vi "GetAvgPatientStayTimeMultipleRooms.vi"(8 "error in":errorcluster, 9 "To":timestamp, 10 "From":timestamp, 11 "Rooms":string[](array[string])) -> (0 "error out":errorcluster, 1 "AvgStayTime(s)":dbl, 2 "TotalNumberOfPatients":i32, 3 "AvgStayTimePerRoom":dbl[](array[numeric]), 5 "NumOfPatientsPerRoom":i32[](array[numeric]))   [LabVIEW 2015, in "DatabaseApi.lvlib"]
uses:
  DatabaseApi.lvlib
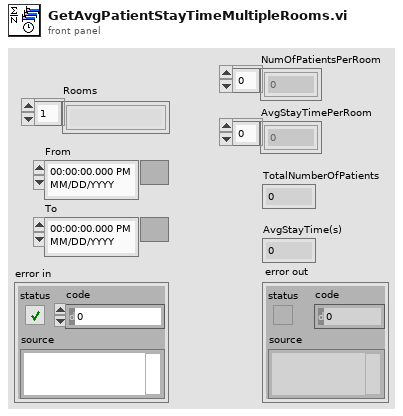
[diagram p1: front panel]
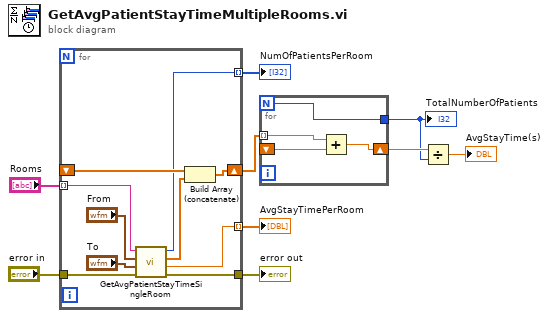
[diagram p0: block diagram]
diagram:
  n1 = for {
    tunnel: "error in" -> [w19]
    tunnel: [w18] -> w6
    tunnel: "Rooms" -> [w15] mode=indexing
    shift-right: [w14] -> w4
    shift-left: _ -> [w13]
    tunnel: [w11] -> w2 mode=indexing
    tunnel: [w10] -> w1 mode=indexing
    n2 = call "GetAvgPatientStayTimeSingleRoom.vi"("error in"=w19, "To"="To", "From"="From", "RoomNumber"=w15) -> ("error out"=w18:errorcluster, "AvgStayTime(s)"=w10:dbl, "PatientStayTime(s)"=w12:dbl[], "NumOfPatients"=w11:i32)  [unwired: 4 in]
    n3 = Build Array (concatenate)(w13, w12) -> (w14:dbl[])
  }
  "error out" <- w6
  "AvgStayTimePerRoom" <- w1
  "NumOfPatientsPerRoom" <- w2
  n4 = for {
    N -> [w21]
    shift-right: [w23] -> w9
    shift-left: _ -> [w22]
    tunnel: [w21] -> w3
    tunnel: w4 -> [w20] mode=indexing
    n5 = Add(x=w20, y=w22) -> (x+y=w23:dbl)
  }
  "TotalNumberOfPatients" <- w3
  n6 = Divide(x=w9, y=w3) -> (x/y=→"AvgStayTime(s)":dbl)
